vi "MB Serial Modbus Data Unit to String.vi"(10 "Modbus Data Unit":T2={"function"=1, "Data"=[]} {"function" items=["Read Discrete Inputs"=2, "Read Coils"=1, "Write Single Coil"=5, "Write Multiple Coils"=15, "Read Input Register"=4, "Read Holding Registers"=3, "Write Single Register"=6, "Write Multiple Registers"=16, "Read/Write Multiple Registers"=23, "Mask Write Register"=22, "Read FIFO Queue"=24, "Read File Record"=20, "Write File Record"=21, "Read Exception Status"=7, "Diagnostic"=8, "Get Com Event Counter"=11, "Get Com Event Log"=12, "Report Slave ID"=17, "Read Device Identification"=43]; "Data" format="%.0x"}, 11 "Serial Parameters":T1 {"Slave Address" format="%.0x"}) -> (3 "String":string)   [LabVIEW 2019, in "NI_modbus_upd.lvlib"]
uses:
  NI_modbus_upd.lvlib
  Ctl/MB Modbus Data Unit.ctl
  Modbus Data Unit (PDU)/Function.ctl
panel:
  # "VI Name: MB Serial Modbus Data Unit to String.vi\nPurpose: Formats the Modbus message to send."
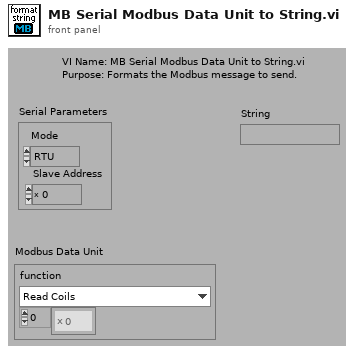
[diagram p1: front panel]
types:
  T1 = cluster{"Mode":enum16{"RTU", "ASCII"}, "Slave Address":u8}
  T2 = typedef "NI_modbus_upd.lvlib/MB Modbus Data Unit.ctl" = cluster{"function":T3, "Data":u8[]}
  T3 = typedef "NI_modbus_upd.lvlib/Function.ctl" = u8
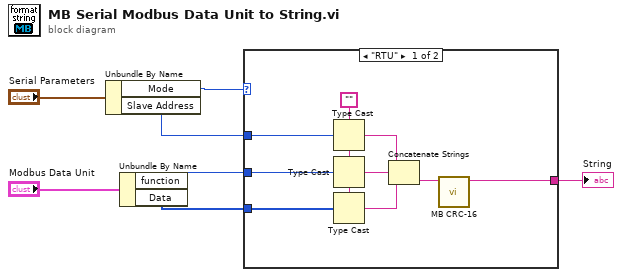
[diagram p0: block diagram]
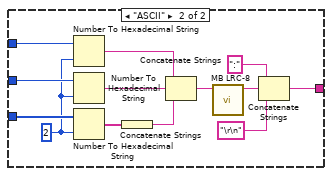
[diagram p2: hidden frame]
diagram:
  n1 = Unbundle By Name("Serial Parameters") -> ("Mode"=w2:enum16{"RTU", "ASCII"}, "Slave Address"=w1:u8)
  n2 = Unbundle By Name("Modbus Data Unit") -> ("function"=w5:T3, "Data"=w4:u8[])
  n3 = case shown="\"RTU\"" w2 {
    tunnel: w1 -> [w13 w29]
    tunnel: w5 -> [w14 w28]
    tunnel: w4 -> [w15 w27]
    tunnel: [w8 w20] -> w7
    frame "RTU" {
      w16 = ""
      n4 = Type Cast(type=w16, x=w13) -> (*(type *) &x=w12:string)
      n5 = Type Cast(type=w16, x=w14) -> (*(type *) &x=w11:string)
      n6 = Type Cast(type=w16, x=w15) -> (*(type *) &x=w10:string)
      n7 = Concatenate Strings(w12, w11, w10) -> (w9:string)
      n8 = call "MB CRC-16.vi"("String"=w9) -> ("String & CRC-16"=w8:string)  [unwired: 8 in, 2 out]
    }
    frame "ASCII" {
      w19 = 2
      n9 = Number To Hexadecimal String(1:w19, 2:w29) -> (0:w26:string)
      n10 = Number To Hexadecimal String(1:w19, 2:w28) -> (0:w25:string)
      n11 = Number To Hexadecimal String(1:w19, 2:w27) -> (0:w18:string[])
      n12 = Concatenate Strings(w18) -> (w17:string)
      n13 = Concatenate Strings(w26, w25, w17) -> (w24:string)
      n14 = call "MB LRC-8.vi"("String"=w24) -> ("string & LRC-8"=w22:string)  [unwired: 8 in, 2 out]
      n15 = Concatenate Strings(":", w22, "\r\n") -> (w20:string)
    }
  }
  "String" <- w7
